vi "Configure Acquisition.vi"(8 "error in (no error)":errorcluster, 11 "Scope PXI Base CFG in":refnum<class "Scope PXI Base CFG.lvclass">) -> (0 "error out":errorcluster, 3 "Scope PXI Base CFG out":refnum<class "Scope PXI Base CFG.lvclass">)   [LabVIEW 2023, in "Scope PXI Base CFG.lvclass"]
uses:
  Scope PXI Base CFG.lvclass
  51f59c3a-b204-4edc-9e9c-c04e48498727.vi
  <vilib>/ErrorRing/Error Ring.xnode
  <vilib>/Utility/error.llb/Error Cluster From Error Code.vi
  Configuration/Configuration JSON/Configuration JSON Base/CFG JSON.lvclass
  D:/git/HAL/HAL GOOP4/Scope/Scope Base CFG/Scope Base CFG.lvclass
  D:/git/HAL/HAL GOOP4/Configuration JSON Base/CFG JSON.lvclass
  D:/git/HAL/HAL GOOP4/Interfaces/IConfigure/IConfigure.lvclass
  D:/git/HAL/HAL GOOP4/Scope/Scope PXI/Base CFG/Scope PXI Base CFG.lvclass
  <instrlib>/niScope/Controls/niScope acquisition type.ctl
panel:
  out "Fetch Relative To":i32(ring)=388 items=["Start"=482, "Trigger"=483, "Pretrigger"=477, "Now"=481, "Read Pointer"=388]
  out "acquisition Type":T1 caption="Acquisition type (Normal)" items=["Normal"=0, "Flex Res"=1, "DDC"=3]
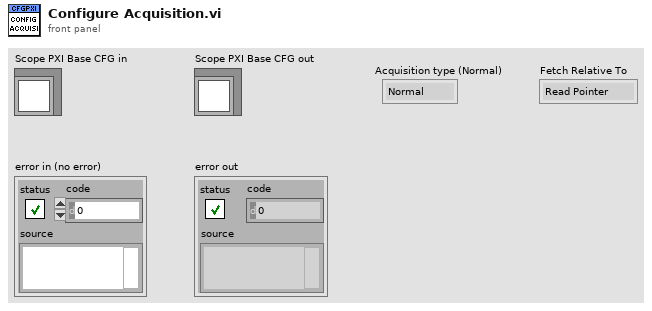
[diagram p1: front panel]
types:
  T1 = typedef "niScope acquisition type.ctl" = i32
  T2 = cluster{"Type":string, "Fetch Relative To":string}
  T3 = typedef "LVStringsAndValuesArrayTypeDef_I32.ctl" = cluster{"String":string, "Value":i32}[]
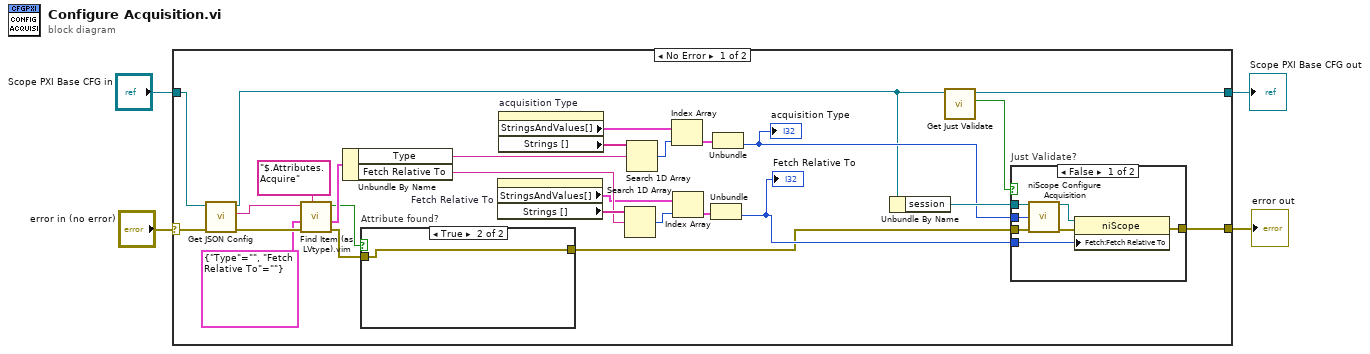
[diagram p0: block diagram]
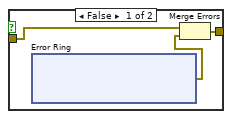
[diagram p3: hidden frame]
diagram:
  n1 = case shown="No Error" "error in (no error)" {
    selector: "error in (no error)" -> [w26 w50]
    tunnel: [w25 w50] -> w3
    tunnel: [w6 w49] -> w1
    tunnel: "Scope PXI Base CFG in" -> [w21 w49]
    frame No Error {
      n2 = call "Get JSON Config.vi"("error in (no error)"=w26, "CFG Base in"=w21) -> ("error out"=w22:errorcluster, "<JSON>Config>"=w19:string, "CFG Base out"=w20:refnum<class "Scope PXI Base CFG.lvclass">)  [unwired: 7 in]
      n3 = call "Find Item (as LVtype).vim"("$Path or Item Name"="$.Attributes.Acquire", "error in (no error)"=w22, "Data Type and Default Value"=T2 {"Type"="", "Fetch Relative To"=""}, "JSON"=w19) -> ("error out"=w8:errorcluster, "Data"=w17:T2, "Found"=w9:bool)  [unwired: 4 in, 1 out]
      n4 = Unbundle By Name(w17) -> ("Type"=w16:string, "Fetch Relative To"=w14:string)
      n5 = case "Attribute found?" shown="True" w9 {
        tunnel: w8 -> [w42 w48]
        tunnel: [w40 w48] -> w7
        frame False {
          n6 = xnode "Error Ring"() -> ("error out"=w41:errorcluster)
          n7 = Merge Errors(w42, w41) -> (w40:errorcluster)
        }
        frame True {
        }
      }
      n8 = property on="Fetch Relative To" class="Ring (strict)"() -> ("StringsAndValues[]"=w12:T3, "Strings []"=w15:string[])  [unwired: 2 in, 2 out]
      n9 = property on="acquisition Type" class="Ring (strict)"() -> ("StringsAndValues[]"=w29:T3, "Strings []"=w30:string[])  [unwired: 2 in, 2 out]
      n10 = Search 1D Array(1D array=w15, element=w14) -> (index of element=w13:i32)  [unwired: 1 in]
      n11 = Search 1D Array(1D array=w30, element=w16) -> (index of element=w28:i32)  [unwired: 1 in]
      n12 = Index Array(array=w29, index=w28) -> (element=w27:cluster{"String":string, "Value":i32})
      n13 = Index Array(array=w12, index=w13) -> (element=w11:cluster{"String":string, "Value":i32})
      n14 = Unbundle(w11) -> ("Value"=w10:i32)  [unwired: 1 out]
      "Fetch Relative To" <- w10
      n15 = Unbundle(w27) -> ("Value"=w23:i32)  [unwired: 1 out]
      "acquisition Type" <- w23
      n16 = Unbundle By Name(w20) -> ("session"=w24:refnum<k15>)
      n17 = call "Get Just Validate.vi"("CFG JSON Base in"=w20) -> ("Just Validate"=w5:bool, "CFG JSON Base out"=w6:refnum<class "Scope PXI Base CFG.lvclass">)  [unwired: 8 in, 1 out]
      n18 = case "Just Validate?" shown="False" w5 {
        tunnel: [w38 w39] -> w25
        tunnel: w24 -> [w37 _]
        tunnel: w23 -> [w36 _]
        tunnel: w10 -> [w35 _]
        tunnel: w7 -> [w32 w39]
        frame False {
          n19 = call <instrlib>:"niScope Configure Acquisition.vi"("instrument handle"=w37, "acquisition Type"=w36, "error in"=w32) -> ("instrument handle out"=w33:refnum<k15>, "error out"=w34:errorcluster)  [unwired: 11 in]
          n20 = property class="niScope"(reference=w33, error in=w34, "Fetch:Fetch Relative To"=w35) -> (error out=w38:errorcluster)  [unwired: 1 out]
        }
        frame True {
        }
      }
    }
    frame Error {
    }
  }
  "error out" <- w3
  "Scope PXI Base CFG out" <- w1
